vi "Mem_StrArray.vi"(8 "error in (no error)":errorcluster, 11 "dataInfo":T1) -> (0 "error out":errorcluster, 2 "SreArray":string[](array[string]))   [LabVIEW 2019, in "Memory Data Access.lvlib"]
uses:
  Memory Data Access.lvlib
  Typedef/memoryDataBlock.ctl
  Global/Global.vi
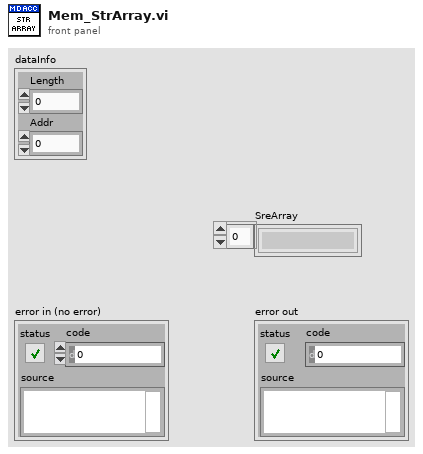
[diagram p1: front panel]
types:
  T1 = typedef "Memory Data Access.lvlib/memoryDataBlock.ctl" = cluster{"Length":u32, "Addr":u64}
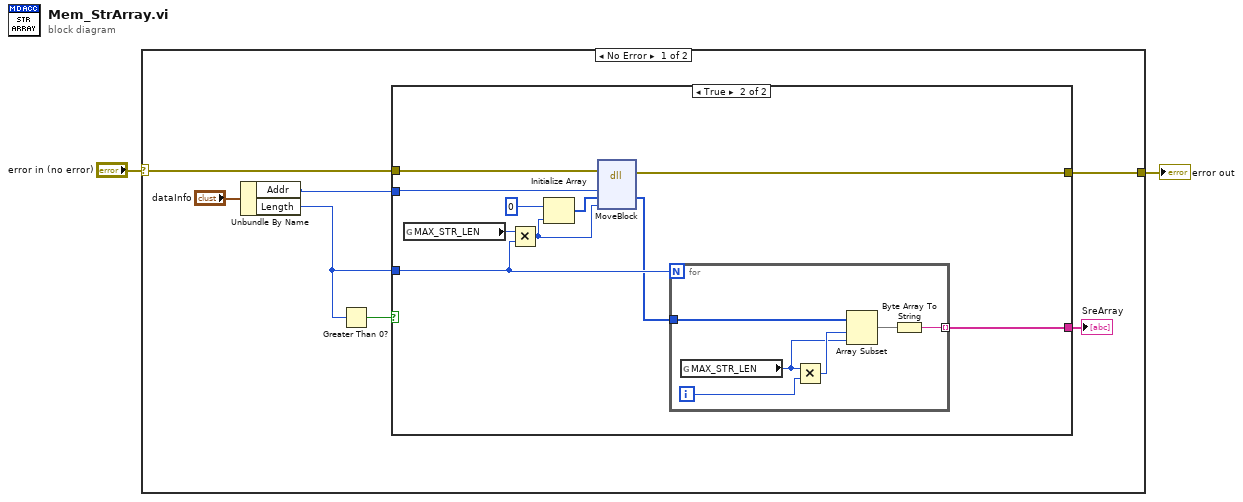
[diagram p0: block diagram]
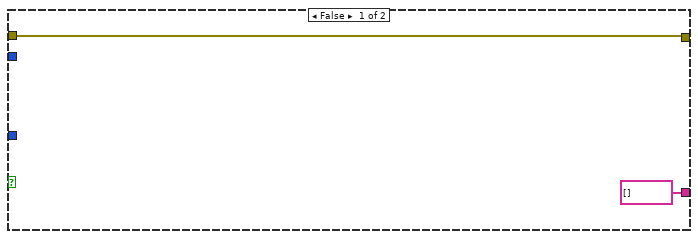
[diagram p2: hidden frame]
diagram:
  n1 = case shown="No Error" "error in (no error)" {
    selector: "error in (no error)" -> [w9 w28]
    tunnel: [w8 w28] -> w1
    frame No Error {
      n2 = Unbundle By Name("dataInfo") -> ("Addr"=w5:u64, "Length"=w4:u32)
      n3 = Greater Than 0?(x=w4) -> (x > 0?=w7:bool)
      n4 = case shown="True" w7 {
        tunnel: w9 -> [w11 w21]
        tunnel: [w11 w13] -> w8
        tunnel: w5 -> [_ w19]
        tunnel: w4 -> [_ w16]
        tunnel: [string[] [] w14] -> w3
        frame False {
        }
        frame True {
          n5 = global read "Global.vi" "MAX_STR_LEN"() -> (w17:u32)
          n6 = Multiply(x=w17, y=w16) -> (x*y=w12:u32)
          n7 = Initialize Array(u8 0, w12) -> (w20:u8[])
          n8 = dll-call lib="LabVIEW" fn="MoveBlock"(error in=w21, "Address"=w19, "Destination"=w20, "Size"=w12) -> (error out=w13:errorcluster, "Destination"=w15:u8[])  [unwired: 5 in, 1 out]
          n9 = for {
            N: w16 -> [_]
            tunnel: w15 -> [w27]
            tunnel: [w22] -> w14 mode=indexing
            i -> [w26]
            n10 = global read "Global.vi" "MAX_STR_LEN"() -> (w24:u32)
            n11 = Multiply(x=w24, y=w26) -> (x*y=w25:u32)
            n12 = Array Subset(array=w27, index=w25, length=w24) -> (w23:u8[])
            n13 = Byte Array To String(unsigned byte array=w23) -> (string=w22:string)
          }
        }
      }
      "SreArray" <- w3
    }
    frame Error {
    }
  }
  "error out" <- w1
